vi "Write panel message (SubVI).vi"(3 "Stop BurnIn":refnum<vi>, 4 "rpm":refnum<vi>, 5 "rpm":bool, 6 "PrintTime":bool=TRUE, 7 "Stop":refnum<vi>, 8 "error in (no error)":errorcluster, 9 "Time to wait":dbl, 10 "Strin":string, 11 "String in":refnum<vi>) -> (0 "error out":errorcluster)   [LabVIEW 2017]
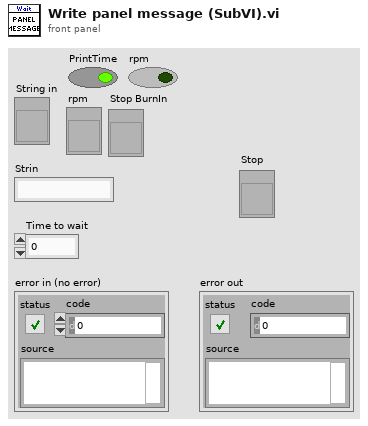
[diagram p1: front panel]
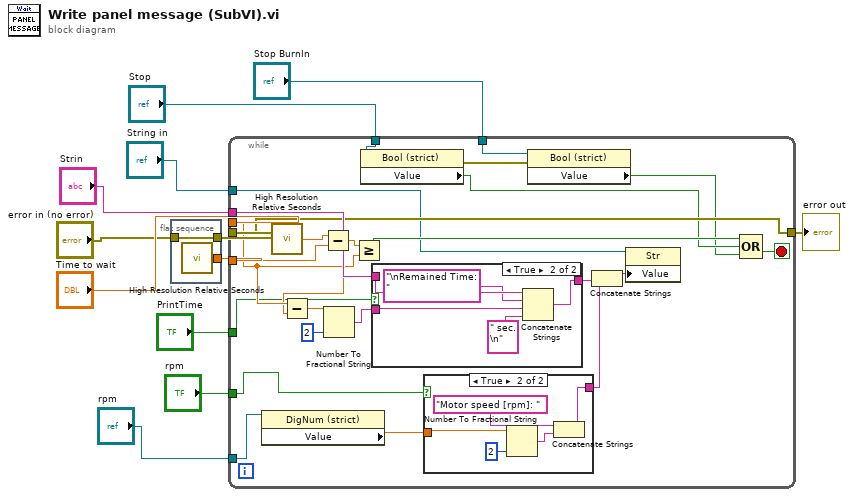
[diagram p0: block diagram]
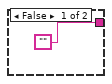
[diagram p2: hidden frame]
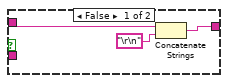
[diagram p3: hidden frame]
diagram:
  n1 = flat-sequence {
    tunnel: [w14] -> w8
    tunnel: "error in (no error)" -> [w14]
    tunnel: [w13] -> w9
    frame #0 {
      n2 = call <vilib>:"High Resolution Relative Seconds.vi"() -> ("relative seconds"=w13:dbl)
    }
  }
  n3 = while {
    tunnel: "Strin" -> [w38]
    tunnel: w8 -> [w33]
    tunnel: w9 -> [w35]
    tunnel: "Time to wait" -> [w29]
    tunnel: [w33] -> w11
    tunnel: "String in" -> [w32]
    tunnel: "Stop" -> [w26]
    tunnel: "PrintTime" -> [w23]
    tunnel: "rpm" -> [w17]
    tunnel: "rpm" -> [w22]
    tunnel: "Stop BurnIn" -> [w18]
    stop <- w25 stop-if-true
    n4 = property class="DigNum (strict)"(reference=w22) -> ("Value"=w21:dbl)  [unwired: 1 in, 2 out]
    n5 = call <vilib>:"High Resolution Relative Seconds.vi"() -> ("relative seconds"=w36:dbl)
    n6 = Subtract(x=w36, y=w35) -> (x-y=w28:dbl)
    n7 = Subtract(x=w29, y=w28) -> (x-y=w30:dbl)
    n8 = Number To Fractional String(number=w30, precision (6)=i16 2) -> (F-format string=w27:string)  [unwired: 2 in]
    n9 = Greater Or Equal?(x=w28, y=w29) -> (x >= y?=w34:bool)
    n10 = property class="Bool (strict)"(reference=w26) -> (error out=w20:errorcluster, "Value"=w24:bool)  [unwired: 1 in, 1 out]
    n11 = case shown="True" w23 {
      tunnel: w38 -> [w47 w52]
      tunnel: [w46 w49] -> w37
      tunnel: w27 -> [_ w48]
      frame False {
        n12 = Concatenate Strings(w47, "\r\n") -> (w46:string)
      }
      frame True {
        n13 = Concatenate Strings(w52, "\nRemained Time: " ("string"), w48, " sec.\n" ("string")) -> (w49:string)
      }
    }
    n14 = case shown="True" w17 {
      tunnel: ["" w41] -> w15
      tunnel: w21 -> [_ w40]
      frame False {
      }
      frame True {
        n15 = Number To Fractional String(number=w40, precision (6)=i16 2) -> (F-format string=w42:string)  [unwired: 2 in]
        n16 = Concatenate Strings("Motor speed [rpm]: " ("string"), w42) -> (w41:string)
      }
    }
    n17 = property class="Bool (strict)"(reference=w18, error in=w20) -> ("Value"=w19:bool)  [unwired: 2 out]
    n18 = Concatenate Strings(w37, w15) -> (w16:string)
    n19 = property class="Str"(reference=w32, "Value"=w16) -> ()  [unwired: 1 in, 2 out]
    n20 = Compound Arithmetic op=OR(w34, w24, w19) -> (w25:bool)
  }
  "error out" <- w11
